vi "main.vi"() -> ()   [LabVIEW 2010]
uses:
  common/xcontrols/XImage/XImage/XImage.xctl
  common/classes/ImageCollection/ImageCollection/ImageCollection.lvclass
  common/classes/Image/Image/Image.lvclass
  <vilib>/Utility/file.llb/Write To Spreadsheet File (string).vi
  <vilib>/Utility/file.llb/Write To Spreadsheet File (DBL).vi
panel:
  in  "button:export":bool
  in  "moving average window size":i32=5
  in  "initial offset":i32=10 min=1
  in  "trace index":i32(slide) min=0 max=39 scale=0.0..39.0
  out "trace":sgl[][](graph)
  in  "no. of sub-points":i32=1 min=1
  in  "button:stop":bool
  in  "XImage":refnum<class "ImageCollection.lvclass">(xcontrol)
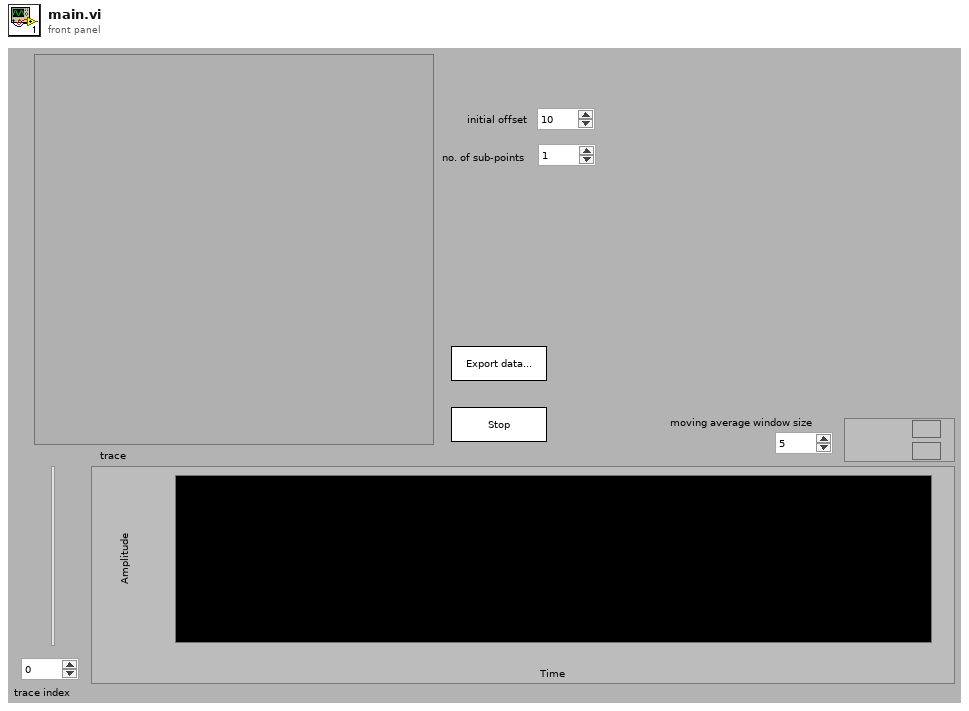
[diagram p1: front panel]
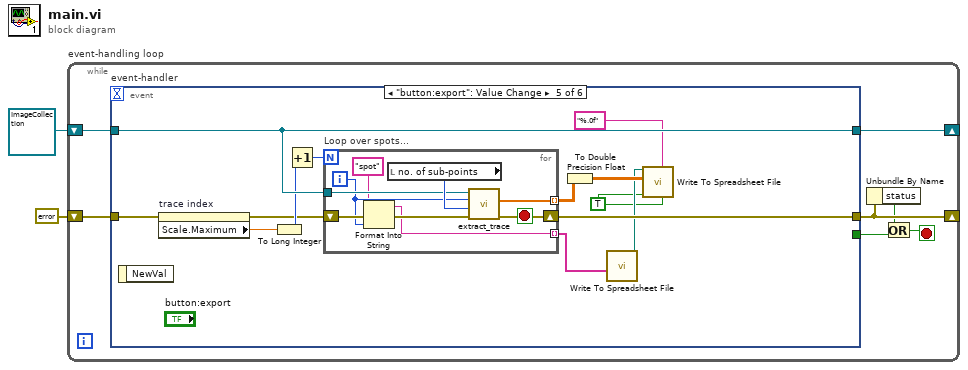
[diagram p0: block diagram]
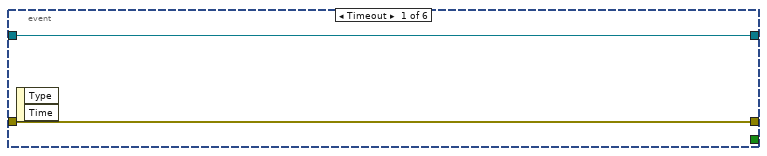
[diagram p2: hidden frame]
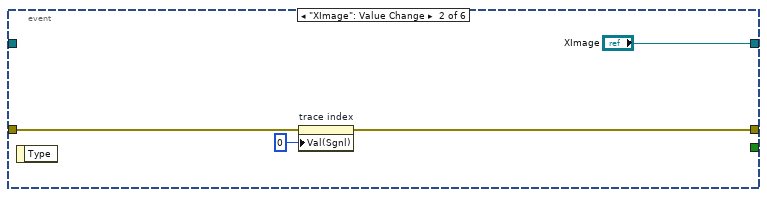
[diagram p3: hidden frame]
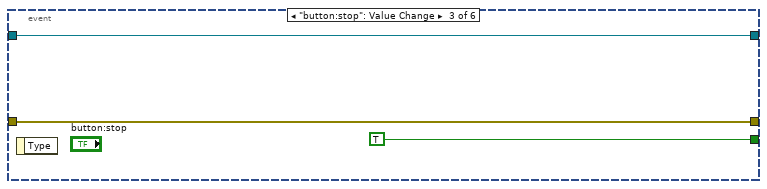
[diagram p4: hidden frame]
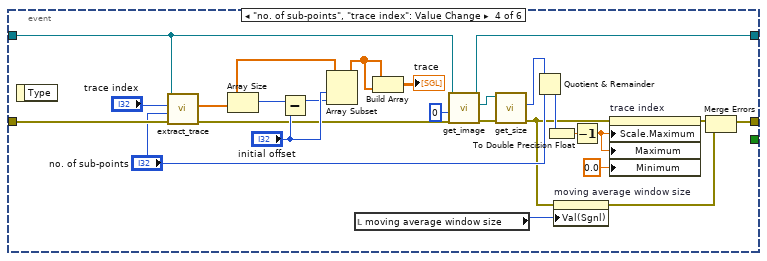
[diagram p5: hidden frame]
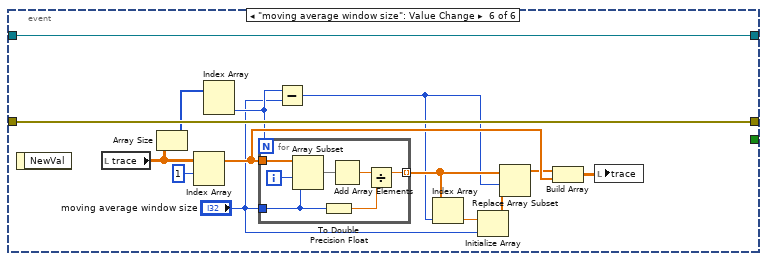
[diagram p6: hidden frame]
diagram:
  n1 = while "event-handling loop" {
    shift-right: [w9] -> _
    shift-left: refnum<class "ImageCollection.lvclass"> refnum ("ImageCollection.lvclass") -> [w8]
    shift-right: [w6] -> _
    shift-left: errorcluster {"status"=FALSE, "code"=0, "source"=""} ("error out") -> [w7]
    stop <- w3 stop-if-true
    n2 = event "event-handler" shown="[4] \"button:export\": Value Change" {
      selector: _ -> [_ _ _ _ _ _]
      dyn-events: _ -> [_ _ _ _ _ _]
      timeout: _ -> [_ _ _ _ _ _]
      tunnel: [w11 "XImage" w18 w32 w55 w79] -> w9
      tunnel: w8 -> [w11 _ w18 w33 w55 w79]
      tunnel: [_ _ TRUE _ _ _] -> w5
      tunnel: w7 -> [w10 w12 w16 w43 w49 w78]
      tunnel: [w10 w14 w16 w20 w56 w78] -> w6
      event Timeout {
        n3 = event-data() -> ()  [unwired: 1 in, 2 out]
      }
      event "XImage": Value Change {
        n4 = event-data() -> ()  [unwired: 1 in, 1 out]
        n5 = property on="trace index" class="Slide (strict)"(error in=w12, "Val(Sgnl)"=0 ("Value (Signaling)")) -> (error out=w14:errorcluster)  [unwired: 1 in, 1 out]
      }
      event "button:stop": Value Change {
        n6 = event-data() -> ()  [unwired: 1 in, 1 out]
      }
      event "no. of sub-points", "trace index": Value Change {
        n7 = event-data() -> ()  [unwired: 1 in, 1 out]
        n8 = call "extract_trace.vi"("error in (no error)"=w43, "sub-pixels per cell"="no. of sub-points", "trace index"="trace index", "ImageCollection in"=w33) -> ("error out"=w34:errorcluster, "traces"=w41:sgl[])  [unwired: 6 in]
        n9 = Array Size(array=w41) -> (size(s)=w40:i32)
        n10 = Subtract(x=w40, y="initial offset") -> (x-y=w38:i32)
        n11 = Array Subset(array=w41, index="initial offset", length=w38) -> (w26:sgl[])
        n12 = local read "moving average window size"() -> (w24:i32)
        n13 = Build Array(w26, w26) -> (→"trace":sgl[][])
        n14 = call-dynamic "get_image.vi"("error in (no error)"=w34, "index"=0, "ImageCollection in"=w33) -> ("error out"=w37:errorcluster, "Image.lvclass"=w35:refnum<class "Image.lvclass">, "ImageCollection out"=w32:refnum<class "ImageCollection.lvclass">)  [unwired: 6 in]
        n15 = call-dynamic "get_size.vi"("error in (no error)"=w37, "Image in"=w35) -> ("error out"=w23:errorcluster, "x resolution"=w31:i32)  [unwired: 2 in, 6 out]
        n16 = Quotient & Remainder(x=w31, y="no. of sub-points") -> (floor(x/y)=w29:i32)  [unwired: 1 out]
        n17 = To Double Precision Float(number=w29) -> (double precision float=w28:dbl)
        n18 = property on="moving average window size" class="DigNum (strict)"(error in=w23, "Val(Sgnl)"=w24) -> (error out=w22:errorcluster)  [unwired: 1 in, 1 out]
        n19 = Decrement(x=w28) -> (x-1=w19:dbl)
        n20 = property on="trace index" class="Slide (strict)"(error in=w23, "Scale.Maximum"=w19, "Maximum"=w19, "Minimum"=0.0 ("Data Entry Limits:Minimum")) -> (error out=w21:errorcluster)  [unwired: 1 in, 1 out]
        n21 = Merge Errors(w21, w22) -> (w20:errorcluster)
      }
      event "button:export": Value Change {
        w44 = TRUE ("transpose? (no:F)")
        n22 = event-data() -> ()  [unwired: 1 in, 1 out]
        n23 = property on="trace index" class="Slide (strict)"(error in=w49) -> (error out=w48:errorcluster, "Scale.Maximum"=w52:dbl)  [unwired: 1 in, 1 out]
        n24 = To Long Integer(number=w52) -> (32bit integer=w50:i32)
        n25 = Increment(x=w50) -> (x+1=w51:i32)
        n26 = for "Loop over spots..." {
          N: w51 -> [_]
          shift-right: [w64] -> w56
          shift-left: w48 -> [w61]
          tunnel: [w63] -> w54 mode=indexing
          tunnel: w55 -> [w62]
          tunnel: [w57] -> w46 mode=indexing
          i -> [w59]
          stop <- w64 stop-if-true
          n27 = Format Into String(initial string="spot", error in=w61, w59) -> (resulting string=w57:string, error out=w60:errorcluster)  [unwired: 1 in]
          n28 = local read "no. of sub-points"() -> (w65:i32)
          n29 = call "extract_trace.vi"("error in (no error)"=w60, "sub-pixels per cell"=w65, "trace index"=w59, "ImageCollection in"=w62) -> ("error out"=w64:errorcluster, "traces"=w63:sgl[])  [unwired: 6 in]
        }
        n30 = To Double Precision Float(number=w54) -> (double precision float=w53:dbl[][])
        n31 = call-poly <vilib>:"Write To Spreadsheet File.vi"("1D data"=w46) -> ("new file path (Not A Path if cancelled)"=w45:path)  [unwired: 7 in]
        n32 = call-poly <vilib>:"Write To Spreadsheet File.vi"("transpose? (no:F)"=w44, "format (%.3f)"="%.0f", "append to file? (new file:F)"=w44, "2D data"=w53, "file path (dialog if empty)"=w45) -> ()  [unwired: 3 in, 1 out]
      }
      event "moving average window size": Value Change {
        n33 = event-data() -> ()  [unwired: 1 in, 1 out]
        n34 = local read "trace"() -> (w75:sgl[][])
        n35 = Array Size(array=w75) -> (size(s)=w74:i32[])
        n36 = Index Array(array=w75, index (row)=1) -> (element=w73:sgl[])  [unwired: 1 in]
        n37 = Index Array(array=w74) -> (element #2=w71:i32)  [unwired: 2 in, 1 out]
        n38 = for {
          N: w71 -> [_]
          tunnel: w73 -> [w86]
          tunnel: "moving average window size" -> [w81]
          tunnel: [w82] -> w70 mode=indexing
          i -> [w85]
          n39 = Array Subset(array=w86, index=w85, length=w81) -> (w84:sgl[])
          n40 = To Double Precision Float(number=w81) -> (double precision float=w80:dbl)
          n41 = Add Array Elements(numeric array=w84) -> (sum=w83:sgl)
          n42 = Divide(x=w83, y=w80) -> (x/y=w82:dbl)
        }
        n43 = Subtract(x=w71, y="moving average window size") -> (x-y=w69:i32)
        n44 = Index Array(array=w70, index=w69) -> (element=w68:dbl)
        n45 = Initialize Array(w68, "moving average window size") -> (w66:dbl[])
        n46 = Replace Array Subset(array=w70, new element=w66, index=w69) -> (w72:dbl[])
        n47 = Build Array(w72, w73) -> (w76:dbl[][])
        n48 = local write "trace"(w76) -> ()
      }
    }
    n49 = Unbundle By Name(w6) -> ("status"=w4:bool)
    n50 = Or(x=w4, y=w5) -> (x .or. y?=w3:bool)
  }
